vi "Init Model Trees.vi"(8 "error in (no error)":errorcluster, 9 "Model to Highlight":string, 10 "SDF Ref":refnum<k24>, 11 "Tree Ref":refnum<k24>) -> (0 "error out":errorcluster)   [LabVIEW 2016, in "System Mapping Tool.lvlib"]
uses:
  System Mapping Tool.lvlib
  NationalInstruments.VeriStand.SystemStorageUI
  NationalInstruments.VeriStand.SystemDefinitionAPI
  NationalInstruments.VeriStand.SystemStorage
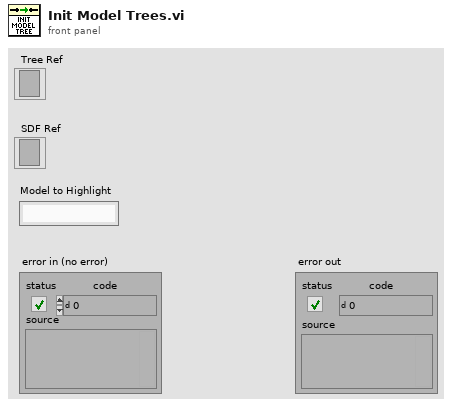
[diagram p1: front panel]
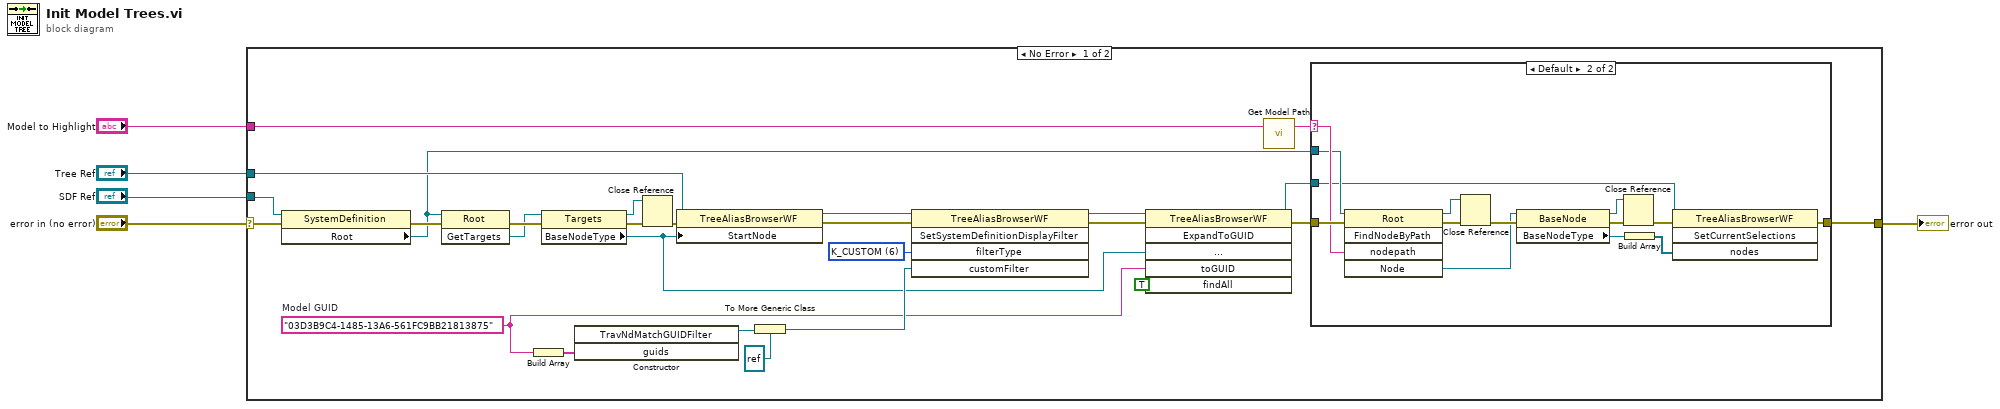
[diagram p0: block diagram]
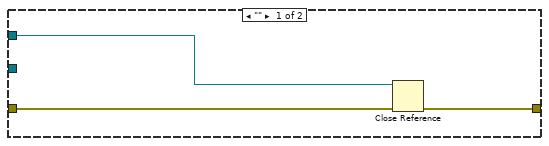
[diagram p2: hidden frame]
diagram:
  n1 = case shown="No Error" "error in (no error)" {
    selector: "error in (no error)" -> [w32 w50]
    tunnel: [w19 w50] -> w4
    tunnel: "SDF Ref" -> [w31 _]
    tunnel: "Tree Ref" -> [w29 _]
    tunnel: "Model to Highlight" -> [w16 _]
    frame No Error {
      w7 = "03D3B9C4-1485-13A6-561FC9BB21813875"  # Model GUID
      w22 = u8 6 items=["K_CHAN_R", "K_CHAN_W", "K_CHAN_RW", "K_CHAN_VOLT", "K_CHAN_FAULT", "K_ALL", "K_CUSTOM", "K_CHAN_R_VIS", "K_CHAN_W_VIS", "K_CHAN_RW_VIS", "K_CHAN_VOLT_VIS", "K_CHAN_FAULT_VIS", "K_WAVE", "K_WAVE_VIS", "K_WAVE_DBL", "K_WAVE_CDB", "K_WAVE_DBL_VIS", "K_WAVE_CDB_VIS"] ("filterType")
      n2 = property class="SystemDefinition"(reference=w31, error in=w32) -> (error out=w30:errorcluster, "Root"=w18:refnum<k24>)  [unwired: 1 out]
      n3 = invoke class="Root" method="GetTargets"(reference=w18, error in=w30) -> (error out=w21:errorcluster, "GetTargets"=w20:refnum<k24>)  [unwired: 1 in, 1 out]
      n4 = Build Array(w7) -> (w13:string[])
      n5 = property class="Targets"(reference=w20, error in=w21) -> (reference out=w26:refnum<k24>, error out=w28:errorcluster, "BaseNodeType"=w6:refnum<k24>)
      n6 = constructor class="TravNdMatchGUIDFilter"("guids"=w13) -> (reference out=w25:refnum<k24>)  [unwired: 3 in, 3 out]
      n7 = Close Reference(reference=w26, error in (no error)=w28) -> (error out=w27:errorcluster)
      n8 = property class="TreeAliasBrowserWF"(reference=w29, error in=w27, "StartNode"=w6) -> (reference out=w15:refnum<k24>, error out=w14:errorcluster)
      n9 = To More Generic Class(target class=refnum<k24> refnum ("customFilter"), reference=w25) -> (generic class reference=w23:refnum<k24>)
      n10 = invoke class="TreeAliasBrowserWF" method="SetSystemDefinitionDisplayFilter"(reference=w15, error in=w14, "filterType"=w22, "customFilter"=w23) -> (reference out=w11:refnum<k24>, error out=w12:errorcluster)  [unwired: 1 in, 3 out]
      n11 = invoke class="TreeAliasBrowserWF" method="ExpandToGUID"(reference=w11, error in=w12, "startNode"=w6, "toGUID"=w7, "findAll"=TRUE) -> (reference out=w9:refnum<k24>, error out=w10:errorcluster)  [unwired: 1 in, 4 out]
      n12 = call "Get Model Path.vi"("Node Path"=w16) -> ("Model Path"=w17:string)  [unwired: 2 in]
      n13 = case shown="Default" w17 {
        selector: w17 -> [_ w48]
        tunnel: w10 -> [w35 w49]
        tunnel: [w34 w42] -> w19
        tunnel: w18 -> [w33 w46]
        tunnel: w9 -> [_ w44]
        frame "" {
          n14 = Close Reference(reference=w33, error in (no error)=w35) -> (error out=w34:errorcluster)
        }
        frame Default {
          n15 = invoke class="Root" method="FindNodeByPath"(reference=w46, error in=w49, "nodepath"=w48) -> (reference out=w45:refnum<k24>, error out=w47:errorcluster, "Node"=w40:refnum<k24>)  [unwired: 2 in, 2 out]
          n16 = Close Reference(reference=w45, error in (no error)=w47) -> (error out=w43:errorcluster)
          n17 = property class="BaseNode"(reference=w40, error in=w43) -> (reference out=w38:refnum<k24>, error out=w41:errorcluster, "BaseNodeType"=w37:refnum<k24>)
          n18 = Close Reference(reference=w38, error in (no error)=w41) -> (error out=w39:errorcluster)
          n19 = Build Array(w37) -> (w36:refnum<k24>[])
          n20 = invoke class="TreeAliasBrowserWF" method="SetCurrentSelections"(reference=w44, error in=w39, "nodes"=w36) -> (error out=w42:errorcluster)  [unwired: 1 in, 3 out]
        }
      }
    }
    frame Error {
    }
  }
  "error out" <- w4
